vi "Raspberry Pi Compatible Compiler for LabVIEW.vi"() -> ()   [LabVIEW 2014]
uses:
  Custom Controls/CompileType.ctl
  RasPi_Services/Download/RuntimeVersion.ctl
  Custom Controls/Local Setup Parameters.ctl
  <vilib>/Platform/browser.llb/Open URL in Default Browser (string).vi
  RasPi_Services/Autodetect/Autodetect.lvlib
  RasPi_Services/Downloader/Downloader.lvclass
  Messaging/SimpleMessaging.lvlib
  RasPi_Services/Download/RasPiDownloader.lvlib
panel:
  in  "exit":bool
  in  "state variables":T2
  in  "Watermark":enum32{"Page 1", "Page 2"}(tab)
  in  "Compile Locally":bool
  out "Animated Image":i16(ring) caption="Ring 2"
  in  "Compilation Type":T3
  in  "Verify Connectivity":bool
  in  "Delete IP":bool
  in  "Edit IP":bool
  in  "Add Ip":bool
  in  "IP List":i32(listbox)
  in  "Blocker":string caption="Status"
  in  "Status":string
  out "Running":bool
  out "VIPath":path caption="Deploy .vi"
  out "StopStat":bool
  in  "FP":bool
  in  "Download":bool
  in  "Help":bool
  in  "Open":bool
  out "Busy":u16(ring)=12
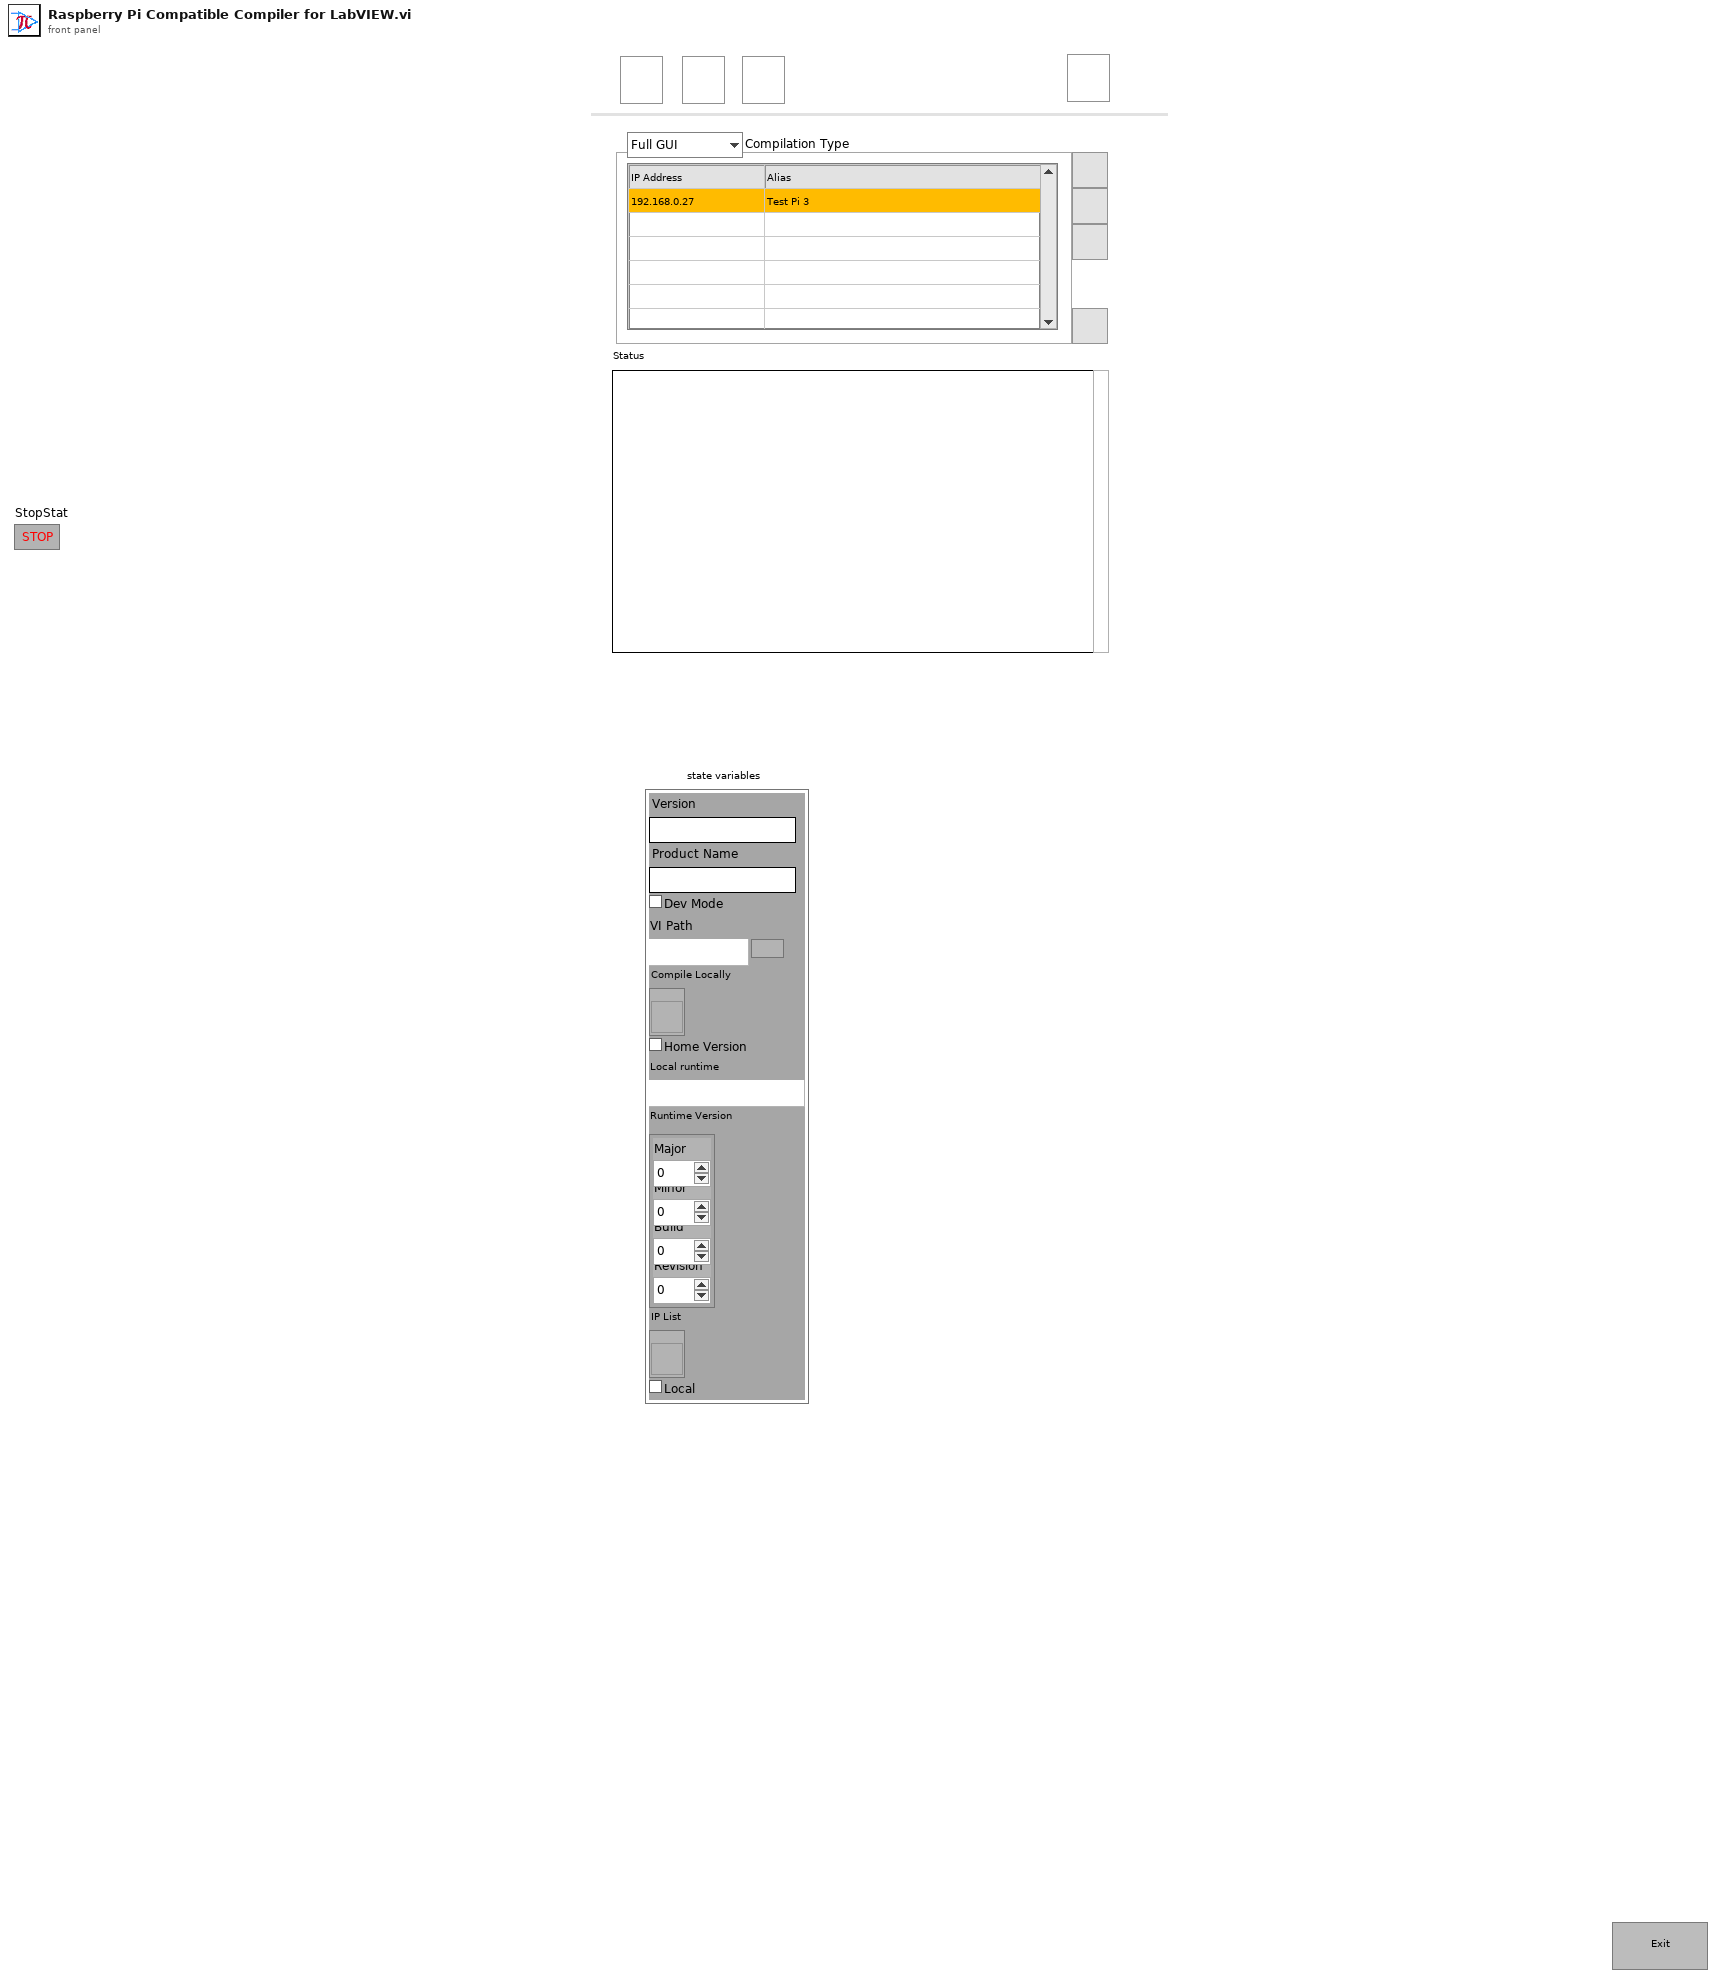
[diagram p1: front panel]
types:
  T1 = typedef "RasPiDownloader.lvlib/RuntimeVersion.ctl" = cluster{"Major":i32, "Minor":i32, "Build":i32, "Revision":i32}
  T2 = cluster{"Version":string, "Product Name":string, "Dev Mode":bool, "VI Path":path, "Compile Locally":refnum<vi>, "Home Version":bool, "Local runtime":path, "Runtime Version":T1, "IP List":refnum<vi>, "Local":bool}
  T3 = typedef "CompileType.ctl" = enum16{"Full GUI", "Console App"}
  T4 = typedef "SimpleMessaging.lvlib/MessageQueueTD.ctl" = refnum<queue>
  T5 = enum8{"Enabled", "Disabled", "Disabled and Grayed Out"}
  T6 = typedef "Local Setup Parameters.ctl" = enum16{"Add Last VI", "Read Last VI", "Add Board IP", "Remove Board IP", "Read All Board IP", "Add Runtime Version", "Read Runtime Version", "Add Package Version", "Read Package Version", "Add VIPCheck Time", "Read VIPCheck Time"}
  T7 = enum16{"Add IP", "Delete IP", "Get IP", "Edit IP"}
  T8 = typedef "Autodetect.lvlib/UDP_Response_TD.ctl" = cluster{"IP address":string, "Port":u16, "response":string}
  T9 = typedef "Autodetect.lvlib/UDP_HostinfoTD.ctl" = cluster{"hostname":string, "version":string}
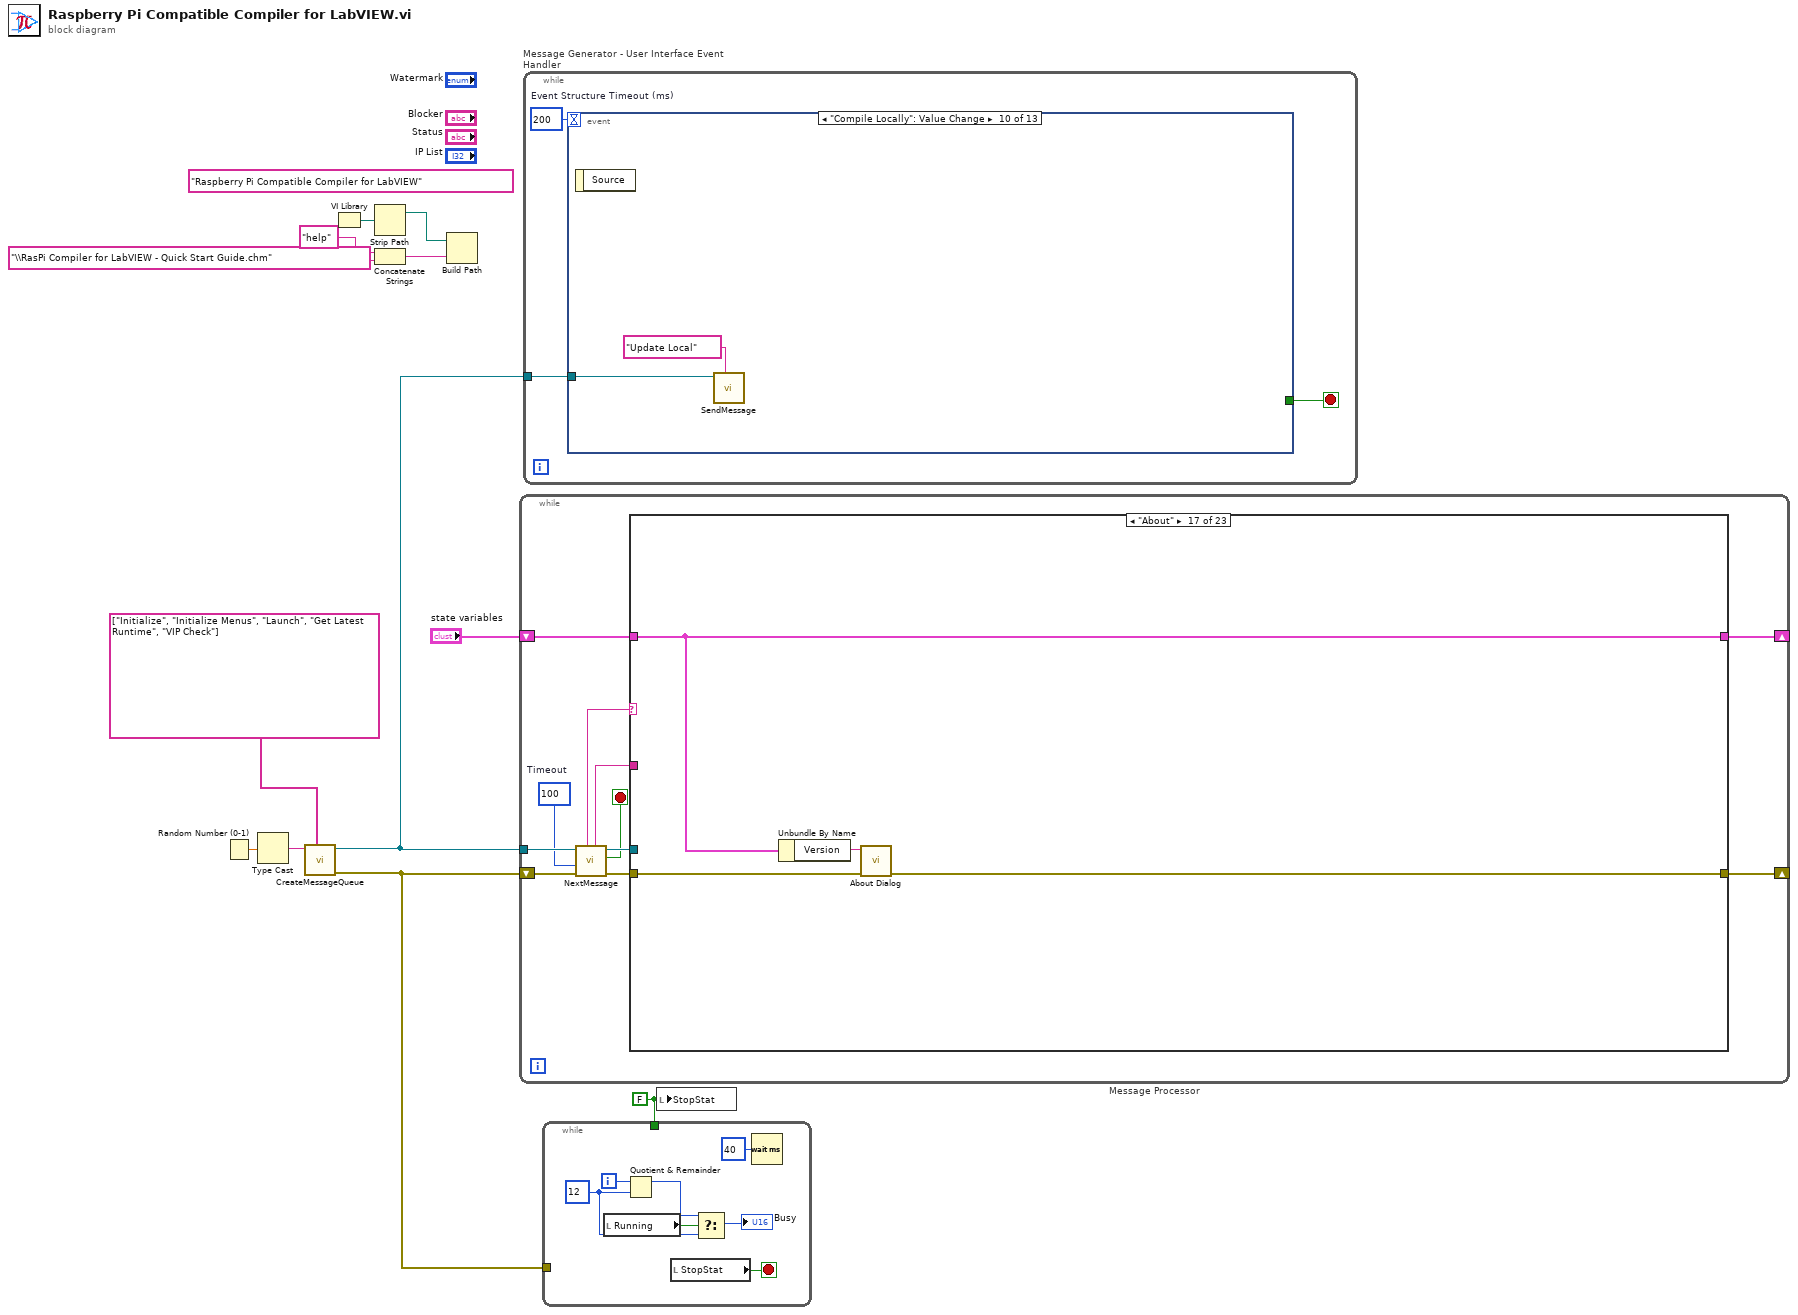
[diagram p0: block diagram]
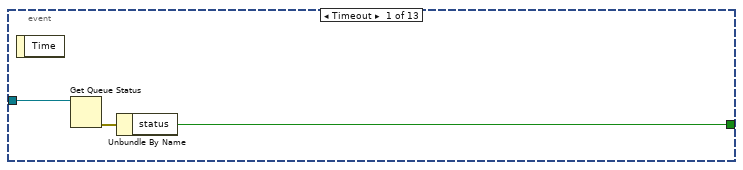
[diagram p2: hidden frame]
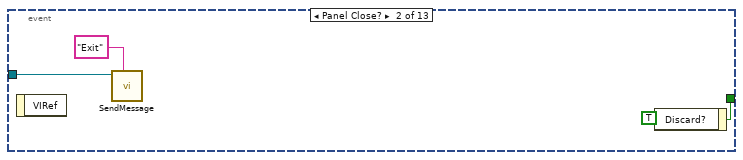
[diagram p3: hidden frame]
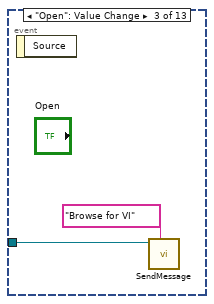
[diagram p4: hidden frame]
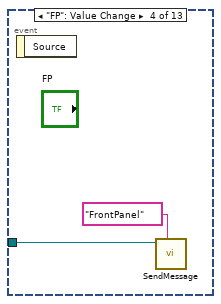
[diagram p5: hidden frame]
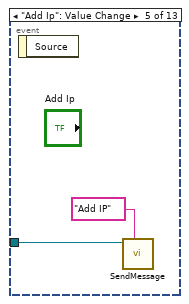
[diagram p6: hidden frame]
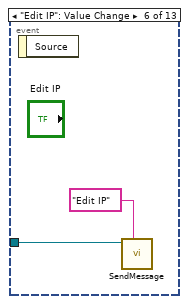
[diagram p7: hidden frame]
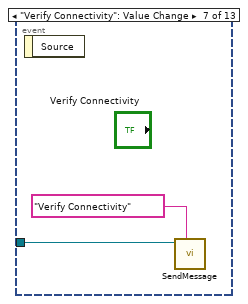
[diagram p8: hidden frame]
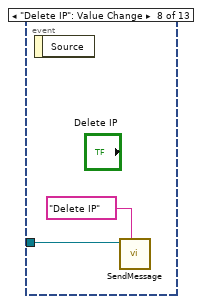
[diagram p9: hidden frame]
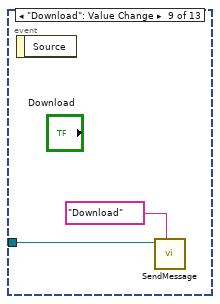
[diagram p10: hidden frame]
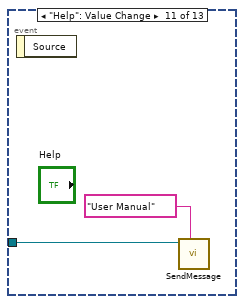
[diagram p11: hidden frame]
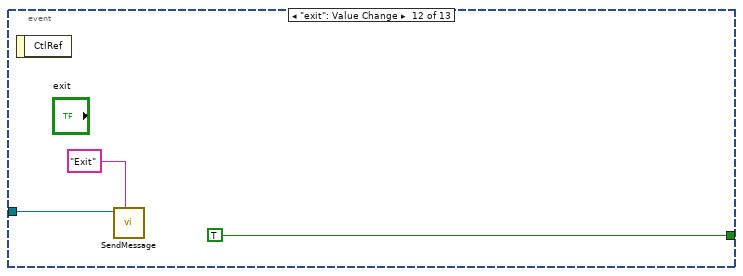
[diagram p12: hidden frame]
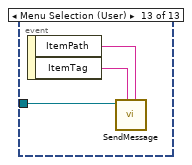
[diagram p13: hidden frame]
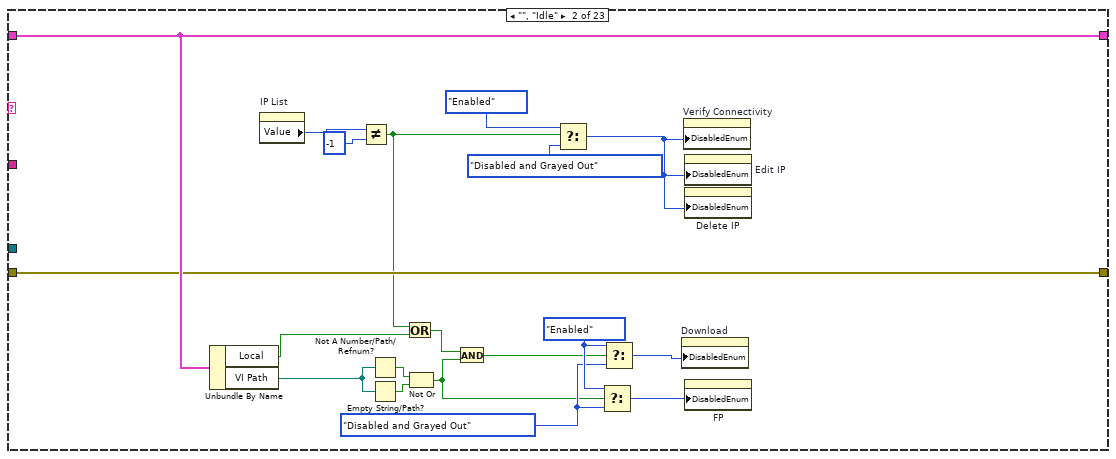
[diagram p15: hidden frame]
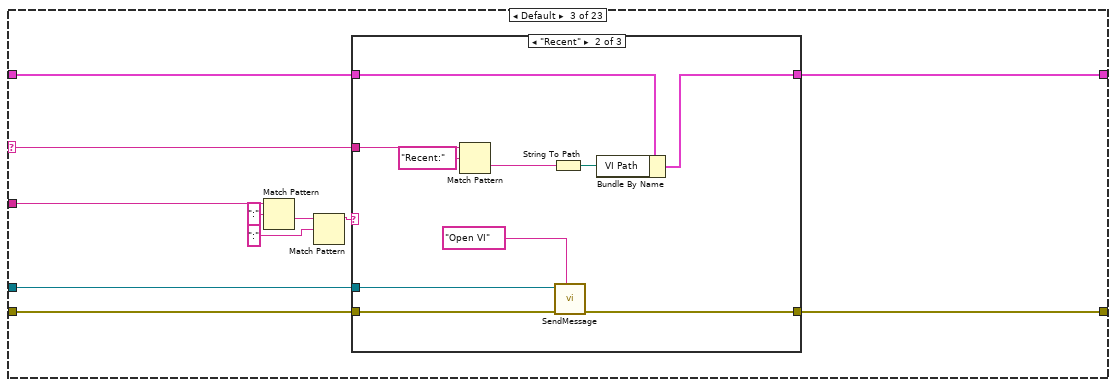
[diagram p16: hidden frame]
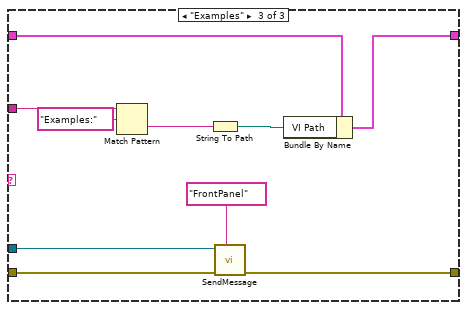
[diagram p18: hidden frame]
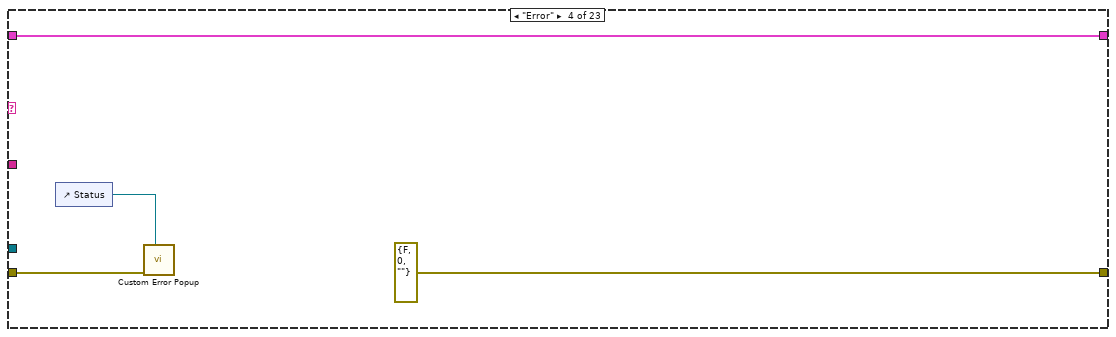
[diagram p19: hidden frame]
diagram:
  w7 = FALSE ("StopStat")
  (unwired) "Raspberry Pi Compatible Compiler for LabVIEW" ("menu tag")
  n1 = Random Number (0-1)() -> (number: 0 to 1=w2:dbl)
  n2 = Type Cast(x=w2) -> (*(type *) &x=w3:string)  [unwired: 1 in]
  n3 = call "CreateMessageQueue.vi"("initial message names"=string[] ["Initialize", "Initialize Menus", "Launch", "Get Latest Runtime", "VIP Check"], "message queue name"=w3) -> ("error out"=w1:errorcluster, "message queue out"=w5:T4)  [unwired: 5 in, 1 out]
  n4 = VI Library() -> (path=w10:path)
  n5 = Strip Path(path=w10) -> (stripped path=w11:path)  [unwired: 1 out]
  n6 = Concatenate Strings("help" ("name or relative path"), "\\RasPi Compiler for LabVIEW - Quick Start Guide.chm" ("name or relative path")) -> (w9:string)
  n7 = Build Path(base path=w11, name or relative path=w9) -> ()  [unwired: 1 out]
  n8 = while "Message Processor" {
    shift-left: w1 -> [w18]
    shift-right: [w21] -> _
    tunnel: w5 -> [w19]
    shift-left: "state variables" -> [w23]
    shift-right: [w22] -> _
    stop <- w13 stop-if-true
    w16 = 100  # Timeout
    n9 = call "NextMessage.vi"("error in"=w18, "timeout in ms (-1)"=w16, "message queue in"=w19) -> ("error out"=w17:errorcluster, "exit"=w13:bool, "message queue out"=w20:T4, "Value"=w14:string, "Name"=w15:string)  [unwired: 1 in, 1 out]
    n10 = case shown="\"About\"" w15 {
      selector: w15 -> [_ _ w51 _ _ _ _ _ _ _ _ _ _ _ _ _ _ _ _ _ _ _ _]
      tunnel: [w25 w35 w46 w81 w83 w108 w111 w128 w176 w212 w226 w234 w236 w237 w272 w305 w318 w323 w336 w356 w391 w403 w408] -> w22
      tunnel: w23 -> [w25 w35 w47 w81 w83 w110 w111 w129 w177 w214 w227 w234 w236 w238 w272 w305 w318 w323 w336 w356 w391 w403 w411]
      tunnel: w20 -> [_ _ w48 _ _ _ _ _ w170 _ _ w232 _ w239 _ _ _ _ _ _ _ _ _]
      tunnel: w17 -> [w24 w34 w50 w79 w82 w92 w114 w131 w179 w216 w225 w233 w235 w241 w275 w306 w321 w325 w339 w358 w395 w401 w412]
      tunnel: [w24 w34 w49 errorcluster {"status"=FALSE, "code"=0, "source"=""} ("error out") w82 w84 w113 _ w169 w209 w225 w228 w235 w240 w274 w307 w320 w324 w337 w357 w393 w400 w405] -> w21
      tunnel: w14 -> [_ _ w45 _ _ _ _ _ w165 _ _ _ _ _ _ _ _ _ _ _ _ _ _]
      frame "---------- Framework Operations ----------" {
      }
      frame "", "Idle" {
        w33 = T5."Disabled and Grayed Out" ("Disabled")
        w38 = T5."Enabled" ("Disabled")
        n11 = Unbundle By Name(w35) -> ("Local"=w26:bool, "VI Path"=w30:path)
        n12 = property on="IP List" class="MCListbox (strict)"() -> ("Value"=w44:i32)  [unwired: 2 in, 2 out]
        n13 = Not Equal?(x=w44, y=-1) -> (x != y?=w31:bool)
        n14 = Not A Number/Path/Refnum?(number/path/refnum=w30) -> (NaN/Path/Refnum?=w28:bool)
        n15 = Empty String/Path?(string/path=w30) -> (empty?=w29:bool)
        n16 = Or(x=w31, y=w26) -> (x .or. y?=w32:bool)
        n17 = Not Or(1:w29, 2:w28) -> (0:w27:bool)
        n18 = And(x=w32, y=w27) -> (x .and. y?=w36:bool)
        n19 = Select(t=T5."Enabled", s=w31, f=T5."Disabled and Grayed Out" ("Disabled")) -> (s? t:f=w40:T5)
        n20 = Select(t=w38, s=w27, f=w33) -> (s? t:f=w37:T5)
        n21 = Select(t=w38, s=w36, f=w33) -> (s? t:f=w39:T5)
        n22 = property on="Download" class="Bool"("DisabledEnum"=w39) -> ()  [unwired: 2 in, 2 out]
        n23 = property on="Verify Connectivity" class="Bool"("DisabledEnum"=w40) -> ()  [unwired: 2 in, 2 out]
        n24 = property on="Edit IP" class="Bool"("DisabledEnum"=w40) -> ()  [unwired: 2 in, 2 out]
        n25 = property on="Delete IP" class="Bool"("DisabledEnum"=w40) -> ()  [unwired: 2 in, 2 out]
        n26 = property on="FP" class="Bool"("DisabledEnum"=w37) -> ()  [unwired: 2 in, 2 out]
      }
      frame Default {
        n27 = Match Pattern(string=w45, regular expression=":") -> (after substring=w53:string)  [unwired: 1 in, 3 out]
        n28 = Match Pattern(string=w53, regular expression=":") -> (before substring=w55:string)  [unwired: 1 in, 3 out]
        n29 = case shown="\"Recent\"" w55 {
          tunnel: w51 -> [_ w66 w76]
          tunnel: w50 -> [w57 w63 w72]
          tunnel: w48 -> [_ w64 w71]
          tunnel: [w57 w62 w73] -> w49
          tunnel: w47 -> [w56 w60 w70]
          tunnel: [w56 w58 w68] -> w46
          frame Default {
          }
          frame "Recent" {
            n30 = Match Pattern(string=w66, regular expression="Recent:") -> (after substring=w65:string)  [unwired: 1 in, 3 out]
            n31 = String To Path(string=w65) -> (path=w59:path)
            n32 = call "SendMessage.vi"("Name"="Open VI" ("Command"), "error in"=w63, "message queue in"=w64) -> ("error out"=w62:errorcluster)  [unwired: 4 in, 2 out]
            n33 = Bundle By Name(cluster=w60, "VI Path"=w59) -> (w58:T2)
          }
          frame "Examples" {
            n34 = Match Pattern(string=w76, regular expression="Examples:") -> (after substring=w75:string)  [unwired: 1 in, 3 out]
            n35 = String To Path(string=w75) -> (path=w69:path)
            n36 = call "SendMessage.vi"("Name"="FrontPanel", "error in"=w72, "message queue in"=w71) -> ("error out"=w73:errorcluster)  [unwired: 4 in, 2 out]
            n37 = Bundle By Name(cluster=w70, "VI Path"=w69) -> (w68:T2)
          }
        }
      }
      frame "Error" {
        n38 = control-ref of="Status"() -> (w78:refnum<vi>)
        n39 = call "Custom Error Popup.vi"("Message Box"=w78, "error in (no error)"=w79) -> ()  [unwired: 9 in, 1 out]
      }
      frame "---------- Generic Operations ----------" {
      }
      frame "Initialize" {
        w85 = FALSE ("Student")
        w89 = FALSE ("Visible")
        n40 = control-ref of="Compile Locally"() -> (w91:refnum<vi>)
        n41 = property on="Watermark" class="TabCtl (strict)"(error in=w92, "Value"=enum32{"Page 1", "Page 2"}."Page 2" ("Watermark")) -> (error out=w98:errorcluster)  [unwired: 1 in, 1 out]
        n42 = property class="Bool (strict)"(reference=w91, error in=w98, "Visible"=w89, "Value"=w89) -> (error out=w87:errorcluster)  [unwired: 1 out]
        n43 = property on="FP" class="Bool"("DisabledEnum"=T5."Disabled and Grayed Out" ("Disabled")) -> ()  [unwired: 2 in, 2 out]
        n44 = Current VI's Menubar() -> (w99:refnum<k9>)
        n45 = Enable Menu Tracking(2:w87, 3:FALSE ("enable (T)"), 4:w99) -> (0:w84:errorcluster)  [unwired: 1 out]
        n46 = property on="IP List" class="MCListbox (strict)"("Value"=-1 ("IP List"), "ItemNames"=string[][] [] ("Item Names")) -> ()  [unwired: 2 in, 2 out]
        n47 = Select(t=enum32{"Page 1", "Page 2"}."Page 1" ("Watermark"), s=w85, f=enum32{"Page 1", "Page 2"}."Page 2") -> (s? t:f=w95:enum32{"Page 1", "Page 2"})
        n48 = property on="Watermark" class="TabCtl (strict)"("Value"=w95) -> ()  [unwired: 2 in, 2 out]
        n49 = property on="Busy" class="Ring (strict)"("Value"=u16 12 ("Busy"), "Visible"=FALSE) -> ()  [unwired: 2 in, 2 out]
        n50 = control-ref of="IP List"() -> (w90:refnum<vi>)
        n51 = local write "StopStat"(FALSE ("StopStat")) -> ()
        n52 = local write "Status"("") -> ()
        n53 = Bundle By Name(cluster=w110, "Product Name"="Raspberry Pi Compatible Compiler for LabVIEW" ("menu tag"), "VI Path"=path "" ("VIPath"), "Compile Locally"=w91, "Dev Mode"=TRUE ("Dev Machine"), "Home Version"=w85, "IP List"=w90) -> (w108:T2)
        "Running" <- FALSE ("Running")
      }
      frame "Initialize Menus" {
        n54 = Current VI's Menubar() -> (w127:refnum<k9>)
        n55 = call "Local Setup Config.vi"("Local Setup Param"=Local_Setup_Parameters."Read Last VI", "error in"=w114) -> ("LastVIs"=w117:string[], "error out"=w116:errorcluster)  [unwired: 10 in, 2 out]
        n56 = Unbundle By Name(w111) -> ("Product Name"=w112:string)
        n57 = call "Update Last VI List to Menu.vi"("LastVIs"=w117, "menu reference"=w127, "error in (no error)"=w116) -> ("error out"=w118:errorcluster)  [unwired: 12 in]
        n58 = call "Local Setup Config.vi"("Local Setup Param"=Local_Setup_Parameters."Read All Board IP", "error in"=w118) -> ("KeyValues"=w121:string[], "KeyNames"=w120:string[], "error out"=w124:errorcluster)  [unwired: 10 in, 1 out]
        n59 = Build Array(w120, w121) -> (w122:string[][])
        n60 = call "Load Examples.vi"("menu reference"=w127, "error in (no error)"=w124, "Release Name"=w112) -> ("error out"=w126:errorcluster)  [unwired: 8 in]
        n61 = Transpose 2D Array(2D array=w122) -> (transposed array=w123:string[][])
        n62 = property on="IP List" class="MCListbox (strict)"("ItemNames"=w123) -> ()  [unwired: 2 in, 2 out]
        n63 = Enable Menu Tracking(2:w126, 3:TRUE ("enable (T)"), 4:w127) -> (0:w113:errorcluster)  [unwired: 1 out]
      }
      frame "Launch" {
        n64 = property class="App"(error in=w131) -> (reference out=w143:refnum<vi>, error out=w144:errorcluster, "App.MenuLaunchVI"=w141:string, "App.MenuLaunchApp"=w142:refnum<vi>)  [unwired: 1 in]
        n65 = Close Reference(reference=w143, error in (no error)=w144) -> (error out=w145:errorcluster)
        n66 = Unbundle By Name(w129) -> ("Product Name"=w130:string)
        n67 = Open VI Reference(application reference (local)=w142, vi path=w141, error in (no error)=w145) -> (vi reference=w138:refnum<vi>, error out=w137:errorcluster)  [unwired: 3 in]
        n68 = property class="VI"(reference=w138, error in=w137) -> (reference out=w140:refnum<vi>, error out=w139:errorcluster, "Path"=w147:path)
        n69 = Close Reference(reference=w140, error in (no error)=w139) -> (error out=w136:errorcluster)
        n70 = Strip Path(path=w147) -> (name=w150:string)  [unwired: 1 out]
        n71 = Empty String/Path?(string/path=w150) -> (empty?=w134:bool)
        n72 = Not Equal?(x=w150, y="GettingStartedWindow.vi") -> (x != y?=w132:bool)
        n73 = Unbundle By Name(w136) -> ("status"=w135:bool)
        n74 = call <vilib>:"Clear Errors.vi"("error in (no error)"=w136) -> ()  [unwired: 5 in, 2 out]
        n75 = Compound Arithmetic op=AND(invert w135, invert w134, w132) -> (w146:bool)
        n76 = case shown="True" w146 {
          tunnel: w147 -> [_ w155]
          tunnel: w130 -> [w153 w160]
          tunnel: w150 -> [_ w159]
          tunnel: [w153 w158] -> w148
          tunnel: [T5."Disabled and Grayed Out" ("Disabled") T5."Enabled" ("Disabled")] -> w149
          tunnel: w129 -> [w151 w156]
          tunnel: [w151 w154] -> w128
          frame False {
          }
          frame True {
            n77 = Bundle By Name(cluster=w156, "VI Path"=w155) -> (w154:T2)
            n78 = Concatenate Strings(w160, " - " ("string"), w159) -> (w158:string)
          }
        }
        n79 = property on="FP" class="Bool"("DisabledEnum"=w149) -> ()  [unwired: 2 in, 2 out]
        n80 = property on="Download" class="Bool"("DisabledEnum"=w149) -> ()  [unwired: 2 in, 2 out]
        n81 = property class="VI"("Front Panel.Title"=w148) -> ()  [unwired: 2 in, 2 out]
      }
      frame "VIP Check" {
        n82 = Scan From String(input string=w165, default 1=FALSE ("Force Check(F)")) -> (error out=w162:errorcluster, output 1=w163:bool)  [unwired: 3 in, 2 out]
        n83 = call <vilib>:"Clear Errors.vi"("error in (no error)"=w162) -> ()  [unwired: 5 in, 2 out]
        n84 = Unbundle By Name(w177) -> ("Product Name"=w178:string, "Home Version"=w175:bool, "Dev Mode"=w166:bool)
        n85 = call "VIP Check.vi"("Dev Mode"=w166, "Force Check(F)"=w163, "error in"=w179, "Home version"=w175, "Product Name"=w178) -> ("error out"=w168:errorcluster, "available version"=w172:string, "Update available"=w173:bool, "Continue"=w174:bool, "Check Version"=w167:bool, "current version"=w171:string)  [unwired: 1 in]
        n86 = case shown="No Error" w168 {
          selector: w168 -> [w181 w208]
          tunnel: w174 -> [w187 _]
          tunnel: w173 -> [w186 _]
          tunnel: w172 -> [w185 _]
          tunnel: w171 -> [w184 w204]
          tunnel: w170 -> [w183 _]
          tunnel: [w182 w203] -> w169
          tunnel: w167 -> [w180 _]
          frame No Error {
            n87 = case shown="False" w187 {
              tunnel: w186 -> [_ _]
              tunnel: w185 -> [_ w200]
              tunnel: w184 -> [_ w199]
              tunnel: w183 -> [w191 _]
              tunnel: w181 -> [w190 w202]
              tunnel: [w189 w202] -> w182
              tunnel: w180 -> [w188 _]
              frame False {
                n88 = case shown="True" w188 {
                  tunnel: w191 -> [_ w195]
                  tunnel: w190 -> [w192 w194]
                  tunnel: [w192 w193] -> w189
                  frame False {
                  }
                  frame True {
                    n89 = call "SendMessage.vi"("Name"="Exit", "error in"=w194, "message queue in"=w195) -> ("error out"=w193:errorcluster)  [unwired: 4 in, 2 out]
                  }
                }
              }
              frame True {
                n90 = local read "Status"() -> (w198:string)
                n91 = Format Into String(format string="A different version is available:\nInstalled : %s\nReleased : %s\n\nNavigate to the Compiler Menu and select Compiler-> Check for Updates to upgrade", initial string=w198, w199, w200) -> (resulting string=w201:string)  [unwired: 1 in, 1 out]
                n92 = local write "Status"(w201) -> ()
              }
            }
          }
          frame Error {
            n93 = call <vilib>:"Clear Errors.vi"("error in (no error)"=w208) -> ("error out"=w203:errorcluster)  [unwired: 5 in, 1 out]
            n94 = local read "Status"() -> (w206:string)
            n95 = Format Into String(format string="Compiler Version Installed : %s\n\nVersion Update Check Couldn't Be Performed as Dev Machine Couldn't Connect to Public Repository", initial string=w206, w204) -> (resulting string=w207:string)  [unwired: 1 in, 1 out]
            n96 = local write "Status"(w207) -> ()
          }
        }
        n97 = Bundle By Name(cluster=w177, "Version"=w171) -> (w176:T2)
      }
      frame "Get Latest Runtime" {
        n98 = call "Runtime Version.vi"("error in"=w216) -> ("error out"=w211:errorcluster, "Runtime Version"=w210:string, "Version"=w215:T1, "Local runtime"=w213:path)  [unwired: 5 in]
        n99 = Bundle By Name(cluster=w214, "Local runtime"=w213, "Runtime Version"=w215) -> (w212:T2)
        n100 = case shown="Error" w211 {
          selector: w211 -> [w217 w223]
          tunnel: w210 -> [_ w219]
          tunnel: [w217 w218] -> w209
          frame No Error {
          }
          frame Error {
            n101 = call <vilib>:"Clear Errors.vi"("error in (no error)"=w223) -> ("error out"=w218:errorcluster)  [unwired: 5 in, 1 out]
            n102 = local read "Status"() -> (w221:string)
            n103 = Format Into String(format string="Runtime Version Installed : %s\n\nVersion Update Check Couldn't Be Performed as Dev Machine Couldn't Connect to Public Repository", initial string=w221, w219) -> (resulting string=w222:string)  [unwired: 1 in, 1 out]
            n104 = local write "Status"(w222) -> ()
          }
        }
      }
      frame "Update Local" {
        n105 = Bundle By Name(cluster=w227, "Local"="Compile Locally") -> (w226:T2)
      }
      frame "Exit" {
        n106 = Release Queue(queue=w232, error in (no error)=w233) -> (error out=w229:errorcluster)  [unwired: 1 in, 2 out]
        n107 = Current VI's Path() -> (path=w231:path)
        n108 = call "Close VI FP.vi"("error in (no error)"=w229, "path"=w231) -> ("error out"=w228:errorcluster)  [unwired: 9 in]
        "StopStat" <- TRUE ("StopStat")
      }
      frame "---------- Application Operations ----------" {
      }
      frame "Browse for VI", "Open" {
        n109 = call "File Dialog2"("error in"=w241, "pattern (all files)"="*.vi") -> ("selected path"=w242:path, "exists"=w243:bool, "error out"=w244:errorcluster)  [unwired: 10 in, 1 out]
        n110 = case shown="True" w243 {
          tunnel: w244 -> [w248 w255]
          tunnel: w242 -> [_ w254]
          tunnel: [w247 w256] -> w240
          tunnel: w239 -> [_ w252]
          tunnel: w238 -> [w246 w250]
          tunnel: [w246 w249] -> w237
          frame False {
            n111 = call <vilib>:"Clear Errors.vi"("error in (no error)"=w248) -> ("error out"=w247:errorcluster)  [unwired: 5 in, 1 out]
          }
          frame True {
            n112 = call "Is VI Runnable.vi"("error in (no error)"=w255, "selected path"=w254) -> ("error out"=w253:errorcluster)  [unwired: 9 in]
            n113 = case shown="No Error" w253 {
              selector: w253 -> [w259 w269]
              tunnel: [w260 w269] -> w256
              tunnel: w254 -> [w262 w268]
              tunnel: w252 -> [w258 _]
              tunnel: [_ w265] -> w251
              tunnel: w250 -> [w263 w264]
              tunnel: [w261 w264] -> w249
              frame No Error {
                n114 = Bundle By Name(cluster=w263, "VI Path"=w262) -> (w261:T2)
                n115 = call "SendMessage.vi"("Name"="Open VI" ("Command"), "error in"=w259, "message queue in"=w258) -> ("error out"=w260:errorcluster)  [unwired: 4 in, 2 out]
              }
              frame Error {
                n116 = Path To String(path=w268) -> (string=w267:string)
                n117 = Format Into String(initial string="Error VI is not runnable\nPath: " ("pattern (all files)"), w267) -> (resulting string=w265:string)  [unwired: 2 in, 1 out]
              }
            }
            n118 = local write "Status"(w251) -> ()
          }
        }
      }
      frame "Open VI" {
        n119 = Unbundle By Name(w272) -> ("Product Name"=w270:string, "VI Path"=w273:path)
        n120 = Current VI's Menubar() -> (w271:refnum<k9>)
        n121 = call "Is VI Runnable.vi"("error in (no error)"=w275, "selected path"=w273) -> ("error out"=w276:errorcluster)  [unwired: 9 in]
        n122 = case shown="No Error" w276 {
          selector: w276 -> [w286 w303]
          tunnel: w270 -> [w296 _]
          tunnel: w271 -> [w283 _]
          tunnel: [w281 w303] -> w274
          tunnel: w273 -> [w291 w302]
          tunnel: [w290 w301] -> w277
          tunnel: ["Loaded: " ("pattern (all files)") "Error Loading: " ("pattern (all files)")] -> w278
          tunnel: [T5."Enabled" ("Disabled") T5."Disabled and Grayed Out" ("Disabled")] -> w280
          frame No Error {
            n123 = Strip Path(path=w291) -> (name=w295:string)  [unwired: 1 out]
            n124 = Path To String(path=w291) -> (string=w290:string)
            n125 = Concatenate Strings(w296, " - " ("string"), w295) -> (w297:string)
            n126 = property class="VI"("Front Panel.Title"=w297) -> ()  [unwired: 2 in, 2 out]
            n127 = Enable Menu Tracking(2:w286, 3:FALSE ("enable (T)"), 4:w283) -> (0:w285:errorcluster)  [unwired: 1 out]
            n128 = call "Local Setup Config.vi"("Local Setup Param"=Local_Setup_Parameters."Add Last VI", "Last VI"=w290, "error in"=w285) -> ("LastVIs"=w292:string[], "error out"=w293:errorcluster)  [unwired: 9 in, 2 out]
            n129 = call "Update Last VI List to Menu.vi"("LastVIs"=w292, "menu reference"=w283, "error in (no error)"=w293) -> ("error out"=w282:errorcluster)  [unwired: 12 in]
            n130 = Enable Menu Tracking(2:w282, 3:TRUE ("enable (T)"), 4:w283) -> (0:w281:errorcluster)  [unwired: 1 out]
          }
          frame Error {
            n131 = Path To String(path=w302) -> (string=w301:string)
          }
        }
        n132 = Format Into String(initial string=w278, w277) -> (resulting string=w279:string)  [unwired: 2 in, 1 out]
        n133 = property on="Download" class="Bool"("DisabledEnum"=w280) -> ()  [unwired: 2 in, 2 out]
        n134 = local write "Status"(w279) -> ()
      }
      frame "FrontPanel" {
        n135 = Unbundle By Name(w305) -> ("VI Path"=w304:path)
        n136 = call "Open VI FP.vi"("error in (no error)"=w306, "VIPath"=w304) -> ("error out"=w308:errorcluster)  [unwired: 9 in]
        n137 = case shown="No Error" w308 {
          selector: w308 -> [w309 _]
          tunnel: [w309 _] -> w307
          tunnel: w304 -> [_ w313]
          frame No Error {
          }
          frame Error {
            n138 = Empty String/Path?(string/path=w313) -> (empty?=w317:bool)
            n139 = Not A Number/Path/Refnum?(number/path/refnum=w313) -> (NaN/Path/Refnum?=w316:bool)
            n140 = Or(x=w316, y=w317) -> (x .or. y?=w315:bool)
            n141 = Format Into String(initial string="Error opening Front Panel\nPath: " ("false string"), w313) -> (resulting string=w311:string)  [unwired: 2 in, 1 out]
            n142 = Append True/False String(1:w315, 2:w311, 3:"No VI loaded" ("true string")) -> (0:w310:string)  [unwired: 1 in]
            n143 = local write "Status"(w310) -> ()
          }
        }
      }
      frame "About" {
        n144 = Unbundle By Name(w318) -> ("Version"=w319:string)
        n145 = call "About Dialog.vi"("error in (no error)"=w321, "SW Version"=w319) -> ("error out"=w320:errorcluster)  [unwired: 9 in]
      }
      frame "Add IP" {
        w329 = "" ("IP Address")
        n146 = Unbundle By Name(w323) -> ("IP List"=w322:refnum<vi>)
        n147 = call "Add IP Address.vi"("error in"=w325, "Alias"=w329, "IP Address"=w329) -> ("error out"=w326:errorcluster, "Alias to Add"=w328:string, "IP to Add"=w327:string)  [unwired: 6 in]
        n148 = call "Edit List.vi"("Method"=enum16{"Add IP", "Delete IP", "Get IP"}."Add IP", "error in (no error)"=w326, "Alias"=w328, "IP Address"=w327, "IP List"=w322) -> ("error out"=w331:errorcluster, "Alias"=w334:string, "IP Address"=w333:string)  [unwired: 3 in, 1 out]
        n149 = call "Local Setup Config.vi"("KeyName"=w333, "Local Setup Param"=Local_Setup_Parameters."Add Board IP", "KeyValue"=w334, "error in"=w331) -> ("error out"=w324:errorcluster)  [unwired: 8 in, 3 out]
      }
      frame "Edit IP" {
        n150 = Unbundle By Name(w336) -> ("IP List"=w335:refnum<vi>)
        n151 = call "Edit List.vi"("Method"=enum16{"Add IP", "Delete IP", "Get IP"}."Get IP", "error in (no error)"=w339, "IP List"=w335) -> ("error out"=w352:errorcluster, "Alias"=w343:string, "IP Address"=w344:string, "Selected Line"=w338:i32)  [unwired: 5 in]
        n152 = call "Add IP Address.vi"("Connected(F)"=TRUE, "error in"=w352, "Alias"=w343, "IP Address"=w344) -> ("error out"=w351:errorcluster, "Alias to Add"=w350:string, "IP to Add"=w349:string)  [unwired: 5 in]
        n153 = call "Edit List.vi"("Selected Line"=w338, "Method"=T7."Edit IP", "error in (no error)"=w351, "Alias"=w350, "IP Address"=w349, "IP List"=w335) -> ("error out"=w353:errorcluster, "Alias"=w341:string, "IP Address"=w342:string)  [unwired: 2 in, 1 out]
        n154 = call "Local Setup Config.vi"("KeyName"=w344, "Local Setup Param"=Local_Setup_Parameters."Remove Board IP", "KeyValue"=w343, "error in"=w353) -> ("error out"=w346:errorcluster)  [unwired: 8 in, 3 out]
        n155 = call "Local Setup Config.vi"("KeyName"=w342, "Local Setup Param"=Local_Setup_Parameters."Add Board IP", "KeyValue"=w341, "error in"=w346) -> ("error out"=w337:errorcluster)  [unwired: 8 in, 3 out]
      }
      frame "Verify Connectivity" {
        n156 = Unbundle By Name(w356) -> ("IP List"=w355:refnum<vi>)
        n157 = call "Edit List.vi"("Method"=enum16{"Add IP", "Delete IP", "Get IP"}."Get IP", "error in (no error)"=w358, "IP List"=w355) -> ("error out"=w367:errorcluster, "IP Address"=w360:string)  [unwired: 5 in, 2 out]
        n158 = local write "Status"("connecting" ("Status")) -> ()
        n159 = Unbundle By Name(w367) -> ("status"=w366:bool)
        n160 = call "Unicast_UDP_message.vi"("message"="*IDN?", "error in"=w367, "address"=w360) -> ("error out"=w362:errorcluster, "response"=w363:T8)  [unwired: 5 in]
        n161 = Not(x=w366) -> (.not. x?=w368:bool)
        n162 = case shown="No Error" w362 {
          selector: w362 -> [w380 w389]
          tunnel: [w373 w390] -> w357
          tunnel: w363 -> [w382 _]
          tunnel: "Connection Couldn't Be Established" ("response") -> [w385 w388]
          tunnel: [w384 w388] -> w371
          tunnel: [FALSE ("Boolean") _] -> w370
          frame No Error {
            n163 = call "ParseHostInfo.vi"("error in"=w380, "response"=w382) -> ("error out"=w379:errorcluster, "Cluster"=w381:cluster{"IP address":string, "host info":T9})  [unwired: 8 in]
            n164 = Unbundle By Name(w381) -> ("host info.hostname"=w378:string, "host info.version"=w375:string)
            n165 = call <vilib>:"Clear Errors.vi"("error in (no error)"=w379) -> ("error out"=w373:errorcluster)  [unwired: 5 in, 1 out]
            n166 = Format Into String(format string="Hostname: %s\nRuntime Version: %s", initial string="Connection Successful\n" ("response"), w378, w375) -> (resulting string=w376:string)  [unwired: 1 in, 1 out]
            n167 = Not Equal?(x=w375, y="") -> (x != y?=w386:bool)
            n168 = Select(t=w376, s=w386, f=w385) -> (s? t:f=w384:string)
          }
          frame Error {
            n169 = call <vilib>:"Clear Errors.vi"("error in (no error)"=w389) -> ("error out"=w390:errorcluster)  [unwired: 5 in, 1 out]
          }
        }
        n170 = Boolean To (0,1)(Boolean=w368) -> (0, 1=→"Animated Image":i16)
        n171 = Boolean To (0,1)(Boolean=w370) -> (0, 1=w369:i16)
        n172 = local write "Animated Image"(w369) -> ()
        n173 = local write "Status"(w371) -> ()
      }
      frame "Delete IP" {
        n174 = Unbundle By Name(w391) -> ("IP List"=w392:refnum<vi>)
        n175 = call "Edit List.vi"("Method"=enum16{"Add IP", "Delete IP", "Get IP"}."Delete IP", "error in (no error)"=w395, "IP List"=w392) -> ("error out"=w394:errorcluster, "Alias"=w399:string, "IP Address"=w398:string)  [unwired: 5 in, 1 out]
        n176 = call "Local Setup Config.vi"("KeyName"=w398, "Local Setup Param"=Local_Setup_Parameters."Remove Board IP", "KeyValue"=w399, "error in"=w394) -> ("error out"=w393:errorcluster)  [unwired: 8 in, 3 out]
      }
      frame "QuickStart", "User Manual" {
        n177 = call-poly <vilib>:"Open URL in Default Browser.vi"("error in (no error)"=w401, "URL"="https://github.com/labviewforRaspi/LabVIEWforRasPi/wiki") -> ("error out"=w400:errorcluster)  [unwired: 4 in, 1 out]
      }
      frame "Download" {
        n178 = flat-sequence {
          tunnel: w411 -> [w417]
          tunnel: w412 -> [w420]
          tunnel: [w419] -> w410
          tunnel: [w417] -> w409
          tunnel: [w418] -> w406
          tunnel: w410 -> [w436]
          tunnel: w409 -> [w429]
          tunnel: [w429] -> w407
          tunnel: w406 -> [w428]
          tunnel: [w423] -> w404
          tunnel: [w457] -> w408
          tunnel: w407 -> [w457]
          tunnel: [w453] -> w405
          tunnel: w404 -> [w453]
          frame #0 {
            w415 = TRUE ("Running")
            n179 = Boolean To (0,1)(Boolean=w415) -> (0, 1=w414:i16)
            n180 = Unbundle By Name(w417) -> ("IP List"=w416:refnum<vi>)
            n181 = local write "Animated Image"(w414) -> ()
            n182 = local write "Running"(w415) -> ()
            n183 = local write "Status"("" ("Status")) -> ()
            n184 = property on="Busy" class="Ring (strict)"("Visible"=TRUE) -> ()  [unwired: 2 in, 2 out]
            n185 = call "Edit List.vi"("Method"=enum16{"Add IP", "Delete IP", "Get IP"}."Get IP", "error in (no error)"=w420, "IP List"=w416) -> ("error out"=w419:errorcluster, "IP Address"=w418:string)  [unwired: 5 in, 2 out]
          }
          frame #1 {
            n186 = Unbundle By Name(w429) -> ("Runtime Version"=w431:T1, "Local runtime"=w430:path)
            n187 = Unbundle By Name(w429) -> ("Local"=w434:bool, "VI Path"=w435:path)
            n188 = Current VI's Path() -> (path=w438:path)
            n189 = Strip Path(path=w438) -> (stripped path=w426:path)  [unwired: 1 out]
            n190 = control-ref of="Status"() -> (w427:refnum<vi>)
            n191 = call "Compile.vi"("LocalCompiledDir"=w426, "Message Box"=w427, "Compilation Type"="Compilation Type", "DevMode"=w434, "error in"=w436, "VI Path"=w435) -> ("error out"=w432:errorcluster, "Source Dir"=w433:path)  [unwired: 4 in]
            n192 = case shown="True" w434 {
              tunnel: w433 -> [w444 w448]
              tunnel: w432 -> [w445 w450]
              tunnel: w431 -> [w443 _]
              tunnel: w430 -> [w442 _]
              tunnel: [w441 w449] -> w425
              tunnel: w428 -> [w440 _]
              tunnel: w427 -> [w439 w447]
              tunnel: w426 -> [_ w446]
              tunnel: [w439 w447] -> w424
              frame False {
                n193 = call "DownloadCode.vi"("Local Version"=w443, "address"=w440, "Local Runtime"=w442, "error in"=w445, "Message Box"=w439, "Python Source"=w444) -> ("error out"=w441:errorcluster)  [unwired: 5 in]
              }
              frame True {
                n194 = call "Downloader.vi"("Message Box"=w447, "error in"=w450, "source"=w448) -> ("error out"=w452:errorcluster, "Downloader out"=w451:refnum<class "Downloader.lvclass">)  [unwired: 7 in]
                n195 = call "DownloadDevMode.vi"("LocalCompiledPath"=w446, "error in"=w452, "Downloader in"=w451) -> ("error out"=w449:errorcluster)  [unwired: 4 in, 2 out]
              }
            }
            n196 = call "Report Error.vi"("error in"=w425, "Status"=w424) -> ("error out"=w423:errorcluster)  [unwired: 9 in]
          }
          frame #2 {
            w454 = FALSE ("Running")
            n197 = Boolean To (0,1)(Boolean=w454) -> (0, 1=w455:i16)
            n198 = local write "Animated Image"(w455) -> ()
            n199 = local write "Running"(w454) -> ()
            n200 = property on="Busy" class="Ring (strict)"("Visible"=FALSE) -> ()  [unwired: 2 in, 2 out]
          }
        }
      }
    }
  }
  n201 = while "Message Generator - User Interface Event Handler" {
    tunnel: w5 -> [w458]
    stop <- w459 stop-if-true
    w460 = 200  # Event Structure Timeout (ms)
    n202 = event shown="[9] \"Compile Locally\": Value Change" {
      selector: _ -> [_ _ _ _ _ _ _ _ _ _ _ _ _]
      dyn-events: _ -> [_ _ _ _ _ _ _ _ _ _ _ _ _]
      timeout: w460 -> [_ _ _ _ _ _ _ _ _ _ _ _ _]
      tunnel: [w461 w466 _ _ _ _ _ _ _ _ _ TRUE ("Discard?") _] -> w459
      tunnel: w458 -> [w462 w464 w467 w470 w471 w473 w475 w477 w479 w481 w483 w485 w489]
      event Timeout {
        n203 = event-data() -> ()  [unwired: 2 out]
        n204 = Get Queue Status(queue=w462) -> (error out=w463:errorcluster)  [unwired: 2 in, 7 out]
        n205 = Unbundle By Name(w463) -> ("status"=w461:bool)
      }
      event Panel Close? {
        w466 = TRUE ("Discard?")
        n206 = event-data() -> ()  [unwired: 2 out]
        n207 = call "SendMessage.vi"("Name"="Exit", "message queue in"=w464) -> ()  [unwired: 5 in, 3 out]
        n208 = event-data("Discard?"=w466) -> ()  [unwired: 1 in, 1 out]
      }
      event "Open": Value Change {
        n209 = event-data() -> ()  [unwired: 2 out]
        n210 = call "SendMessage.vi"("Name"="Browse for VI", "message queue in"=w467) -> ()  [unwired: 5 in, 3 out]
      }
      event "FP": Value Change {
        n211 = event-data() -> ()  [unwired: 2 out]
        n212 = call "SendMessage.vi"("Name"="FrontPanel", "message queue in"=w470) -> ()  [unwired: 5 in, 3 out]
      }
      event "Add Ip": Value Change {
        n213 = event-data() -> ()  [unwired: 2 out]
        n214 = call "SendMessage.vi"("Name"="Add IP", "message queue in"=w471) -> ()  [unwired: 5 in, 3 out]
      }
      event "Edit IP": Value Change {
        n215 = event-data() -> ()  [unwired: 2 out]
        n216 = call "SendMessage.vi"("Name"="Edit IP", "message queue in"=w473) -> ()  [unwired: 5 in, 3 out]
      }
      event "Verify Connectivity": Value Change {
        n217 = event-data() -> ()  [unwired: 2 out]
        n218 = call "SendMessage.vi"("Name"="Verify Connectivity", "message queue in"=w475) -> ()  [unwired: 5 in, 3 out]
      }
      event "Delete IP": Value Change {
        n219 = event-data() -> ()  [unwired: 2 out]
        n220 = call "SendMessage.vi"("Name"="Delete IP", "message queue in"=w477) -> ()  [unwired: 5 in, 3 out]
      }
      event "Download": Value Change {
        n221 = event-data() -> ()  [unwired: 2 out]
        n222 = call "SendMessage.vi"("Name"="Download", "message queue in"=w479) -> ()  [unwired: 5 in, 3 out]
      }
      event "Compile Locally": Value Change {
        n223 = event-data() -> ()  [unwired: 2 out]
        n224 = call "SendMessage.vi"("Name"="Update Local", "message queue in"=w481) -> ()  [unwired: 5 in, 3 out]
      }
      event "Help": Value Change {
        n225 = event-data() -> ()  [unwired: 2 out]
        n226 = call "SendMessage.vi"("Name"="User Manual", "message queue in"=w483) -> ()  [unwired: 5 in, 3 out]
      }
      event "exit": Value Change {
        n227 = event-data() -> ()  [unwired: 2 out]
        n228 = call "SendMessage.vi"("Name"="Exit", "message queue in"=w485) -> ()  [unwired: 5 in, 3 out]
      }
      event Menu Selection (User) {
        n229 = event-data() -> ("ItemPath"=w490:string, "ItemTag"=w488:string)  [unwired: 1 out]
        n230 = call "SendMessage.vi"("Value"=w490, "Name"=w488, "message queue in"=w489) -> ()  [unwired: 4 in, 3 out]
      }
    }
  }
  n231 = while {
    tunnel: w7 -> [_]
    tunnel: w1 -> [_]
    i -> [w495]
    stop <- w497 stop-if-true
    w492 = u32 12 ("y")
    n232 = local read "Running"() -> (w494:bool)
    n233 = Quotient & Remainder(x=w495, y=w492) -> (x-y*floor(x/y)=w493:u32)  [unwired: 1 out]
    n234 = local read "StopStat"() -> (w497:bool)
    n235 = Select(t=w493, s=w494, f=w492) -> (s? t:f=→"Busy":u32)
    n236 = Wait (ms)(milliseconds to wait=u32 40) -> ()  [unwired: 1 out]
  }
  n237 = local write "StopStat"(w7) -> ()
